vi "Vi Element.vi"(8 "Fehler (in)":errorcluster caption="Fehlerkonstante", 10 "Element Beschriftiung":string, 11 "VI Referenz":refnum<vi>) -> (0 "Fehler (out)":errorcluster caption="Fehlerkonstante", 3 "Elem Referenz":refnum<vi>)   [LabVIEW 2020, in "allgemeine Sub-VIs.lvlib"]
doc: "Sucht ein Element nach seiner Bezeichnung in einer VI über die VI Referenz und gibt eine Elementreferenz zurück.\nRIW 25.04.2018"
uses:
  allgemeine Sub-VIs.lvlib
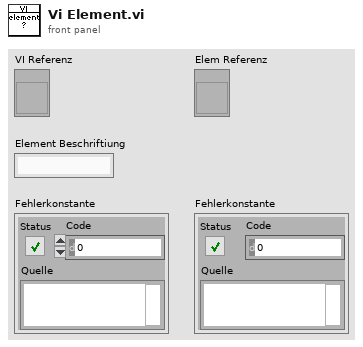
[diagram p1: front panel]
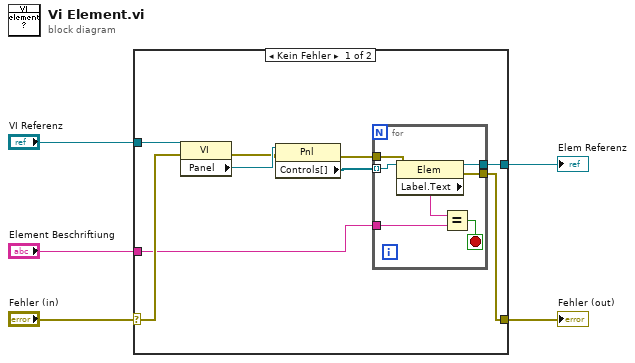
[diagram p0: block diagram]
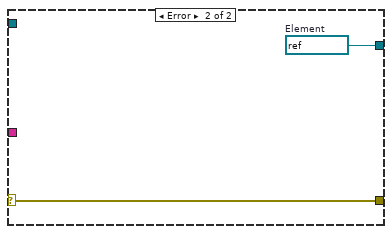
[diagram p2: hidden frame]
diagram:
  n1 = case shown="Kein Fehler" "Fehler (in)" {
    selector: "Fehler (in)" -> [w13 w23]
    tunnel: [w6 w23] -> w4
    tunnel: "VI Referenz" -> [w14 _]
    tunnel: "Element Beschriftiung" -> [w9 _]
    tunnel: [w8 w22] -> w2
    frame No Error {
      n2 = property class="VI"(reference=w14, error in=w13) -> (error out=w11:errorcluster, "Panel"=w12:refnum<vi>)  [unwired: 1 out]
      n3 = property class="Pnl"(reference=w12, error in=w11) -> (error out=w7:errorcluster, "Controls[]"=w10:refnum<vi>[])  [unwired: 1 out]
      n4 = for {
        tunnel: w10 -> [w21] mode=indexing
        tunnel: w9 -> [w19]
        tunnel: [w17] -> w8
        tunnel: w7 -> [w16]
        tunnel: [w15] -> w6
        stop <- w18 stop-if-true
        n5 = property class="Elem"(reference=w21, error in=w16) -> (reference out=w17:refnum<vi>, error out=w15:errorcluster, "Label.Text"=w20:string)
        n6 = Equal?(x=w20, y=w19) -> (x = y?=w18:bool)
      }
    }
    frame Error {
      w22 = refnum<vi> refnum  # Element
    }
  }
  "Fehler (out)" <- w4
  "Elem Referenz" <- w2
